vi "TwGetSegmentProfileFromH5.vi"(2 "segmentProfile in":sgl[](array[numeric]), 3 "error in (no error)":errorcluster, 4 "writeIndex":i32, 5 "bufIndex":i32, 6 "peakIndex":i32, 7 "filename":string) -> (0 "segmentProfile out":sgl[](array[numeric]), 1 "error out":errorcluster)   [LabVIEW 2009]
uses:
  TwH5Dll.dll
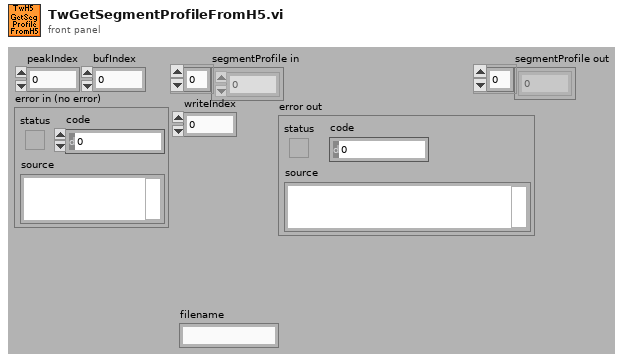
[diagram p1: front panel]
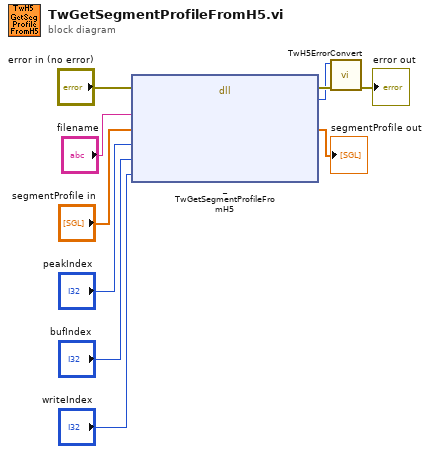
[diagram p0: block diagram]
diagram:
  n1 = dll-call lib="C:/src/85_TofDaq_current/DllWrappers/LabView/TwH5Dll/TwH5Dll.dll" fn="_TwGetSegmentProfileFromH5"(error in="error in (no error)", "filename"="filename", "segmentProfile"="segmentProfile in", "peakIndex"="peakIndex", "bufIndex"="bufIndex", "writeIndex"="writeIndex") -> (error out=w9:errorcluster, "TwRetVal"=w8:i32, "segmentProfile"=→"segmentProfile out":sgl[])  [unwired: 6 in, 1 out]
  n2 = call "TwH5ErrorConvert.vi"("error in (no error)"=w9, "error code"=w8) -> ("error out"=→"error out":errorcluster)  [unwired: 9 out]
